vi "Run (ARGB with Mask).vi"(7 "OCR Level (Default: Word)":T6, 8 "error in (no error)":errorcluster, 9 "Greyscale Mask in":T1, 10 "ARGB Image in":T5, 11 "Text Tesseract in":refnum<class "Text Tesseract.lvclass">) -> (0 "error out":errorcluster, 1 "Detections":T2[](array[typedef]), 2 "Detected Text":string, 3 "Text Tesseract":refnum<class "Text Tesseract.lvclass">)   [LabVIEW 2020, in "feature_detection.lvlib" / "Text Tesseract.lvclass"]
uses:
  Text Tesseract.lvclass
  Text Tesseract.lvclass/Text Tesseract.ctl
  d21e2b8c-d7dd-47ce-9b78-18a6692dbbcb.vi
  OCR Level.ctl
  image/ARGB Image.ctl
  image/image.lvlib
  Rectangle Corners.ctl
  Detection Result.ctl
  common/Image Point (Integer).ctl
  common/common.lvlib
  image/Greyscale Image.ctl
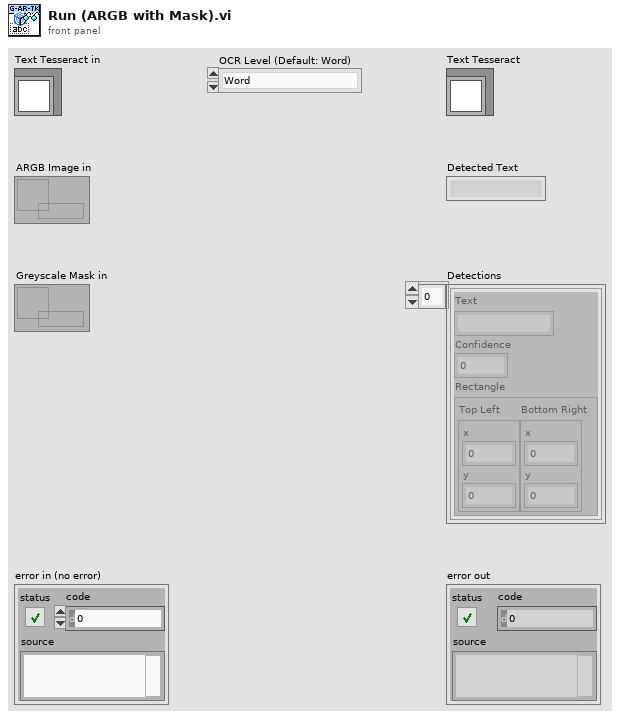
[diagram p1: front panel]
types:
  T1 = typedef "image.lvlib/Greyscale Image.ctl" = refnum<data-value>
  T2 = typedef "feature_detection.lvlib/Text Tesseract.lvclass/Detection Result.ctl" = cluster{"Text":string, "Confidence":sgl, "Rectangle":T3}
  T3 = typedef "feature_detection.lvlib/Text Tesseract.lvclass/Rectangle Corners.ctl" = cluster{"Top Left":T4, "Bottom Right":T4}
  T4 = typedef "common.lvlib/Image Point (Integer).ctl" = cluster{"x":i32, "y":i32}
  T5 = typedef "image.lvlib/ARGB Image.ctl" = refnum<data-value>
  T6 = typedef "feature_detection.lvlib/Text Tesseract.lvclass/OCR Level.ctl" = enum16{"Word", "Line"}
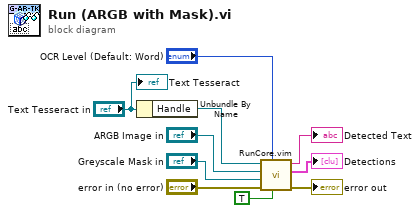
[diagram p0: block diagram]
diagram:
  n1 = Unbundle By Name("Text Tesseract in") -> ("Handle"=w10:refnum<data-value>)
  n2 = call "RunCore.vim"("Has Mask?"=TRUE, "OCR Level"="OCR Level (Default: Word)", "error in (no error)"="error in (no error)", "Mask"="Greyscale Mask in", "ARGB Image in"="ARGB Image in", "Handle"=w10) -> ("error out"=→"error out":errorcluster, "Detections"=→"Detections":T2[], "Detected Text"=→"Detected Text":string)  [unwired: 3 in]
  "Text Tesseract" <- "Text Tesseract in"
